vi "Nichtlineares Pendelmodell mit I.vi"(0 "Kraft (N)":dbl, 1 "Position_t0":dbl, 2 "Winkel_t0":dbl, 3 "Winkelg._t0":dbl) -> (7 "Position":dbl, 8 "Geschwindigkeit":dbl, 9 "Winkel":dbl, 10 "Winkelgesch":dbl)   [LabVIEW 2014]
uses:
  <vilib>/Simulation/Implementation/Shared/SIMSCR Execution Mode.ctl
  <vilib>/Simulation/Scripting/Companion Diagram/SimConfigNode/SimParams.ctl
  <vilib>/Simulation/Scripting/Companion Diagram/SimConfigNode/_simSolvers.ctl
  <vilib>/Simulation/Param Hierarchy/Typedefs/SIMPH Param Control Actions.ctl
  <vilib>/Simulation/Implementation/Shared/SIM limit type.ctl
  <vilib>/Simulation/Implementation/Shared/NILVSim_ParamChanged.vi
  <vilib>/Simulation/Implementation/Shared/NILVSIM_BeginStep.vi
  <vilib>/Simulation/ContinuousLinear/Implementation/NILVSim Integrator new.llb/SIM Integrator distributor (scalar).vi
  <vilib>/Simulation/ContinuousLinear/Implementation/NILVSim Integrator new.llb/SIM Integrator collector (scalar).vi
  <vilib>/Simulation/Implementation/Shared/NILVSim_Manager.vi
  <vilib>/Utility/error.llb/Clear Errors.vi
  <vilib>/Simulation/Implementation/Shared/NILVSim_FinalizeModel.vi
  <vilib>/Simulation/Implementation/Shared/SIM Unbundle Sim Info.vi
  <vilib>/Simulation/Implementation/Shared/SIMSH Read Queue.vi
  <vilib>/Simulation/Implementation/Shared/NILVSim_Initialize.vi
  <vilib>/Simulation/Utility/Implementation/NILVSim Get Time and IsAcceptedStep.vi
  <vilib>/Simulation/Implementation/Shared/NILVSim_GetModelError.vi
  <vilib>/Simulation/Implementation/Shared/SIM SimErrorHandler.vi
  <vilib>/Simulation/Implementation/Shared/SIM Bundle Sim Info.vi
  <vilib>/Simulation/Scripting/Companion Diagram/SimConfigNode/SimDog.xnode
  <vilib>/Simulation/Implementation/XNodeFramework/SimXNode/SimX.xnode
  <vilib>/Simulation/ContinuousLinear/Implementation/NILVSim Integrator new.llb/SIM Integrator (scalar).vi
  <vilib>/Simulation/Implementation/Shared/NI_SIM_Implementation.lvlib
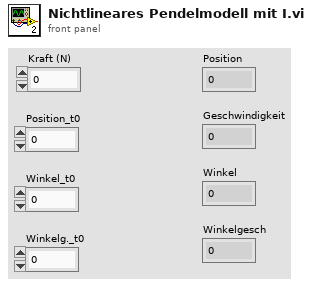
[diagram p1: front panel]
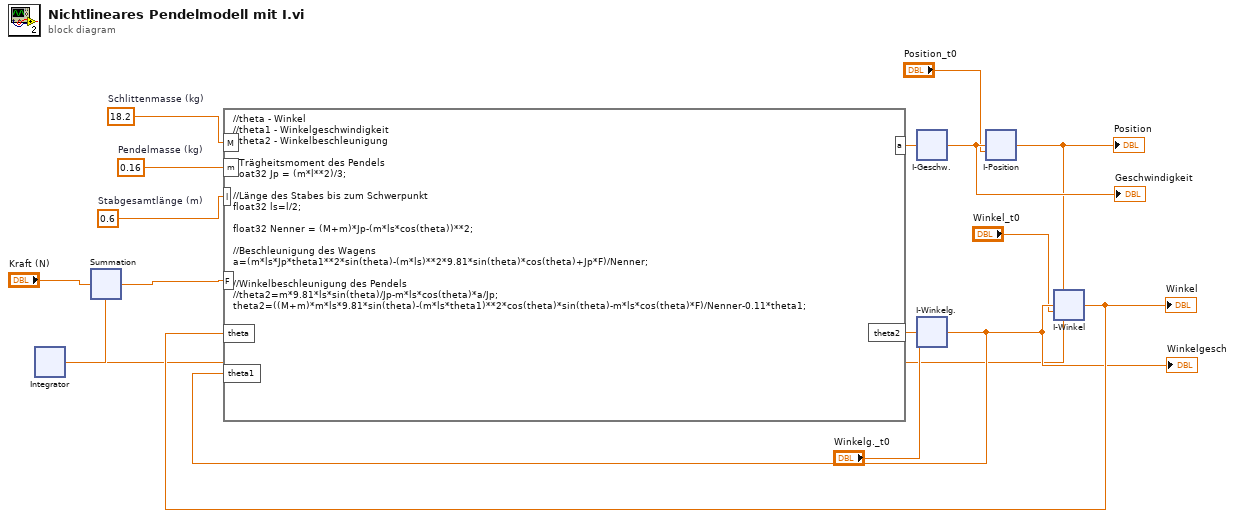
[diagram p0: block diagram]
diagram:
  w6 = 0.6  # Stabgesamtlänge (m)
  w9 = 0.16  # Pendelmasse (kg)
  w12 = 18.2  # Schlittenmasse (kg)
  n1 = xnode "Integrator"("input"=w1) -> ("output"=w2:dbl)  [unwired: 9 in, 2 out]
  n2 = xnode "Summation"("Operand1"="Kraft (N)", "Operand2"=w2) -> ("Result"=w3:dbl)
  n3 = formula code="//theta - Winkel\n//theta1 - Winkelgeschwindigkeit\n//theta2 - Winkelbeschleunigung\n\n//Trägheitsmoment des Pendels\nfloat32 Jp = (m*l**2)/3;\n\n//Länge des Stabes bis zum Schwerpunkt\nfloat32 ls=l/2;\n\nfloat32 Nenner = (M+m)*Jp-(m*ls*cos(theta))**2;\n\n//Beschleunigung des Wagens\na=(m*ls*Jp*theta1**2*sin(theta)-(m*ls)**2*9.81*sin(theta)*cos(theta)+Jp*F)/Nenner;\n\n//Winkelbeschleunigung des Pendels\n//theta2=m*9.81*ls*sin(theta)/Jp-m*ls*cos(theta)*a/Jp;\ntheta2=((M+m)*m*ls*9.81*sin(theta)-(m*ls*theta1)**2*cos(theta)*sin(theta)-m*ls*cos(theta)*F)/Nenner-0.11*theta1;" ("Formelknoten")("M"=w12, "m"=w9, "l"=w6, "theta"=w15, "theta1"=w14, "F"=w3) -> ("a"=w7:dbl, "theta2"=w8:dbl)
  n4 = xnode "I-Geschw."("input"=w7) -> ("output"=w13:dbl)  [unwired: 9 in, 2 out]
  "Geschwindigkeit" <- w13
  n5 = xnode "I-Winkelg."("input"=w8, "initial condition"="Winkelg._t0") -> ("output"=w14:dbl)  [unwired: 8 in, 2 out]
  "Winkelgesch" <- w14
  n6 = xnode "I-Position"("input"=w13, "initial condition"="Position_t0") -> ("output"=w1:dbl)  [unwired: 8 in, 2 out]
  "Position" <- w1
  n7 = xnode "I-Winkel"("input"=w14, "initial condition"="Winkel_t0") -> ("output"=w15:dbl)  [unwired: 8 in, 2 out]
  "Winkel" <- w15
